vi "USB - Write and Read a Synchronous Message.vi"(8 "error in":errorcluster, 10 "Message to Send":string, 11 "VISA resource name in":refnum<visa-resource-name>) -> (0 "error out":errorcluster, 2 "Received Text":string, 3 "VISA resource name out":refnum<visa-resource-name>)   [LabVIEW 2021]
doc: "Send a USB/Serial message and listen for the response. \nThe linefeed character is used to detect the end of the response message."
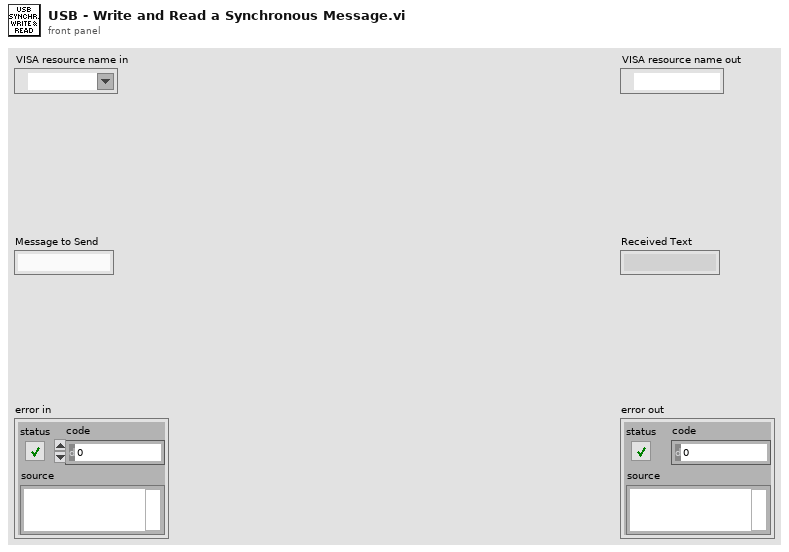
[diagram p1: front panel]
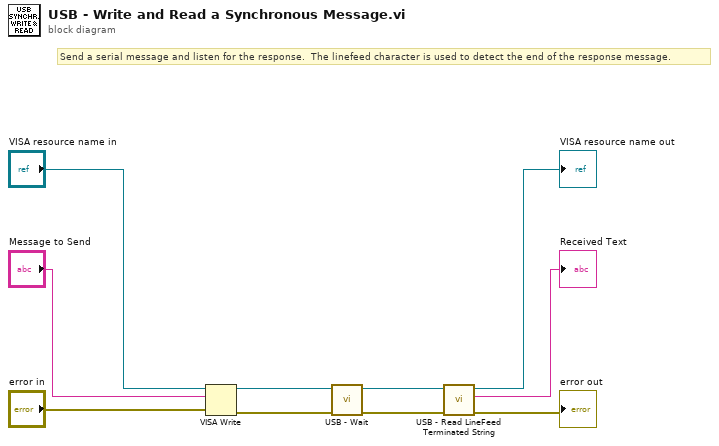
[diagram p0: block diagram]
diagram:
  # "Send a serial message and listen for the response.  The linefeed character is used to detect the end of the response message."
  n1 = VISA Write(VISA resource name="VISA resource name in", write buffer="Message to Send", error in (no error)="error in") -> (VISA resource name out=w3:refnum<visa-resource-name>, error out=w9:errorcluster)  [unwired: 1 out]
  n2 = call "USB - Wait.vi"("error in"=w9, "VISA Resource Name In"=w3) -> ("error out"=w8:errorcluster, "VISA Resource Name Out"=w2:refnum<visa-resource-name>)  [unwired: 8 in]
  n3 = call "USB - Read LineFeed Terminated String.vi"("error in"=w8, "VISA resource name in"=w2) -> ("error out"=→"error out":errorcluster, "Received Text"=→"Received Text":string, "VISA resource name out"=→"VISA resource name out":refnum<visa-resource-name>)  [unwired: 7 in]
